vi "GT Get Axis Enc Vel Filter.vi"(8 "error in (no error)":errorcluster caption="错误输入（无错误）", 9 "pFilterNumExp":i16[](array[numeric]), 10 "axis":i16, 11 "cardNum":i16) -> (0 "error out":errorcluster caption="错误输出", 1 "pFilterNumExp out":i16[](array[numeric]), 3 "function return":i16)   [LabVIEW 2014, in "gts.lvlib"]
doc: "GT_API GT_GetAxisEncVelFilter(short cardNum,short axis,short *pFilterNumExp);"
uses:
  gts.lvlib
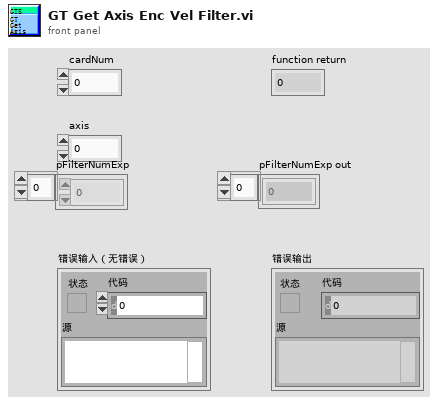
[diagram p1: front panel]
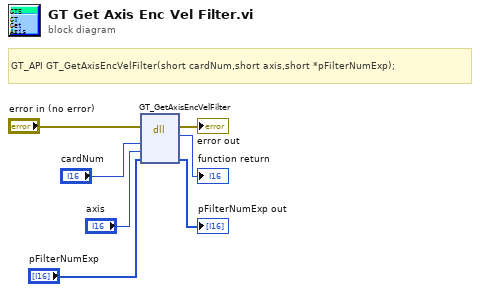
[diagram p0: block diagram]
diagram:
  # "GT_API GT_GetAxisEncVelFilter(short cardNum,short axis,short *pFilterNumExp);"
  n1 = dll-call lib="PTH2habs D固高科技资料GTS控制卡GTS卡18年上半年资料dllVC32bit\nmulti_cardgts.*" fn="GT_GetAxisEncVelFilter"(error in="error in (no error)", "cardNum"="cardNum", "axis"="axis", "pFilterNumExp"="pFilterNumExp") -> (error out=→"error out":errorcluster, "返回类型"=→"function return":i16, "pFilterNumExp"=→"pFilterNumExp out":i16[])  [unwired: 4 in, 1 out]
